vi "GetClassTemplateMethods.vi"(0 "MethodTemplatePath":path, 5 "error in":errorcluster) -> (6 "InterfaceMethodNames":string[](array[string]), 8 "InterfaceMethodPaths":path[](array[path]), 10 "NormalMethodNames":string[](array[string]), 11 "PropertyNodeMethodPaths":path[](array[path]), 12 "NormalMethodPaths":path[](array[path]), 13 "PropertyNodeMethodNames":string[](array[string]), 15 "OverrideMethodNames":string[](array[string]), 16 "OverrideMethodPaths":path[](array[path]), 17 "PropertyMethodNames":string[](array[string]), 18 "PropertyMethodPaths":path[](array[path]), 19 "error out":errorcluster)   [LabVIEW 2020, in "ClassWriterNative.lvclass"]
uses:
  <resource>/Framework/Providers/Open_GDS/ClassProviders/Provider_LvNativeClass/ClassWriterNative_class/ClassWriterNative.lvclass
  <vilib>/Utility/config.llb/Read Key (Path).vi
  <vilib>/Utility/config.llb/NI_LVConfig.lvlib
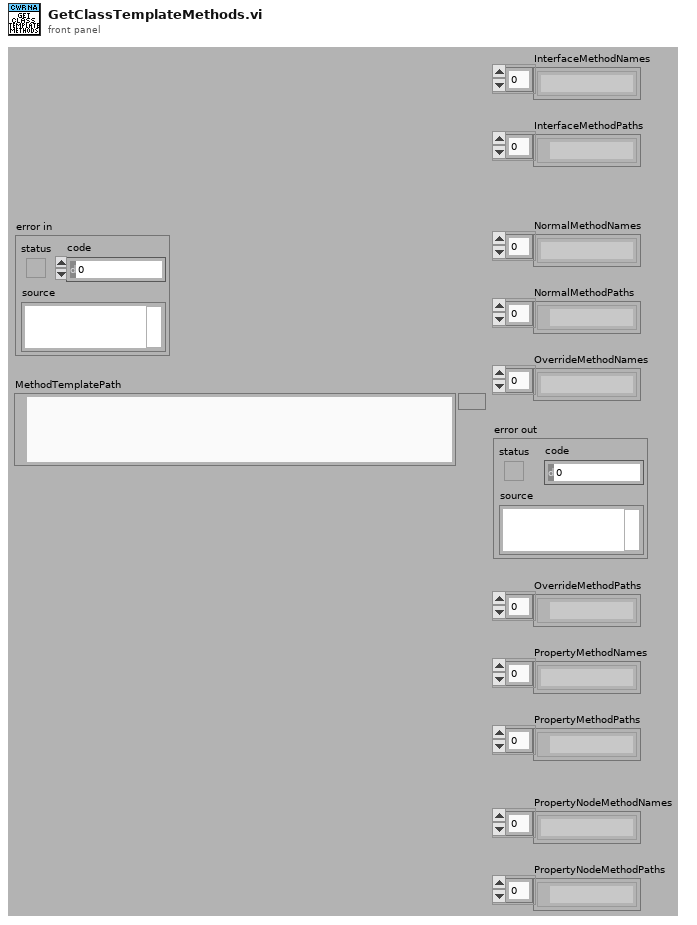
[diagram p1: front panel]
types:
  T1 = typedef "NI_LVConfig.lvlib/Config Data RefNum.ctl" = refnum<k1>
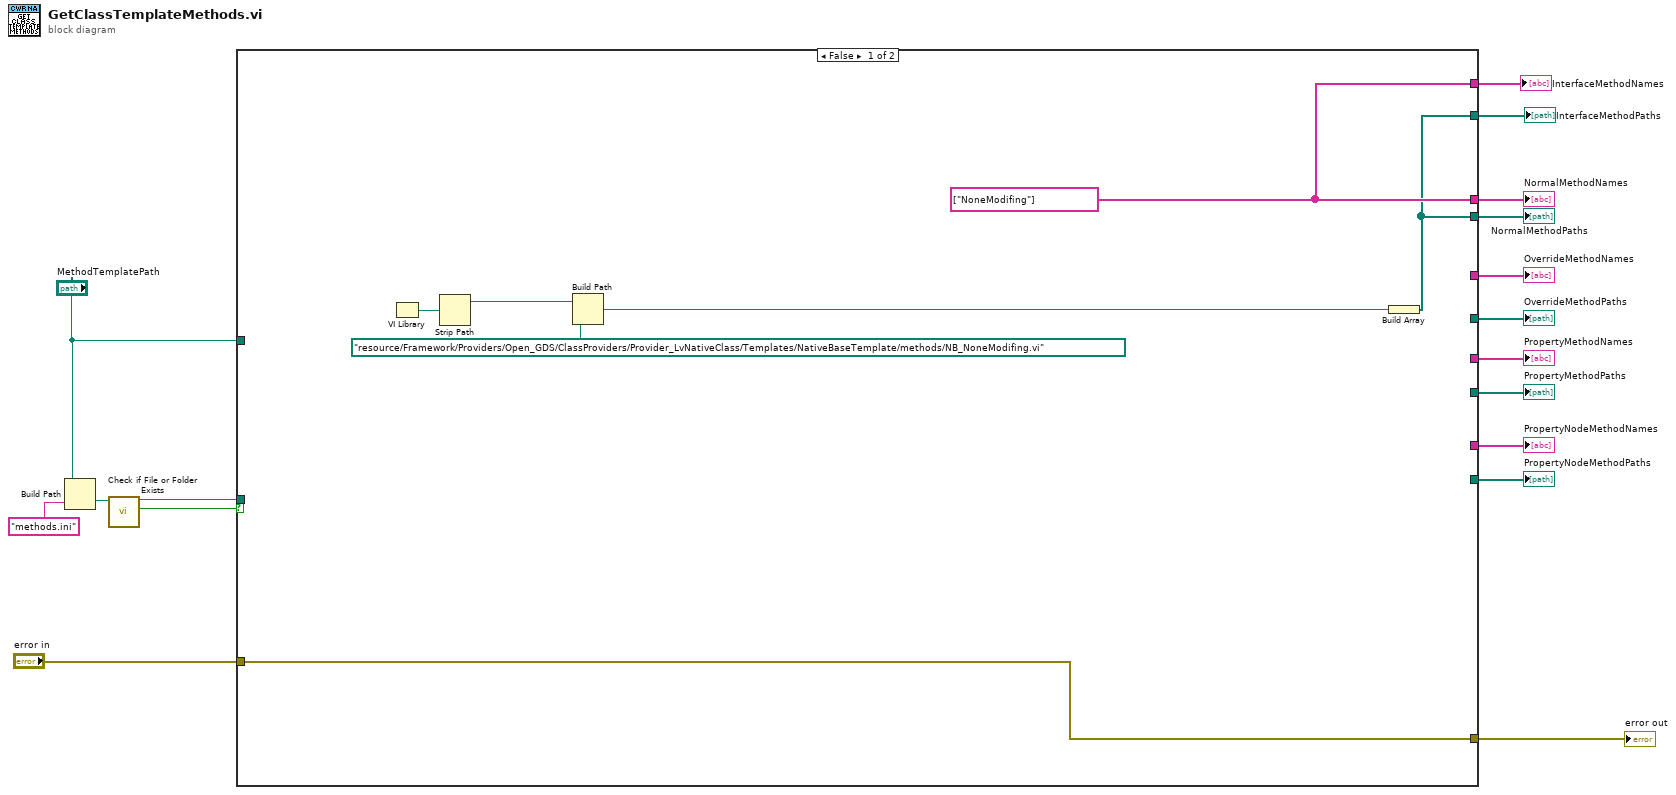
[diagram p0: block diagram]
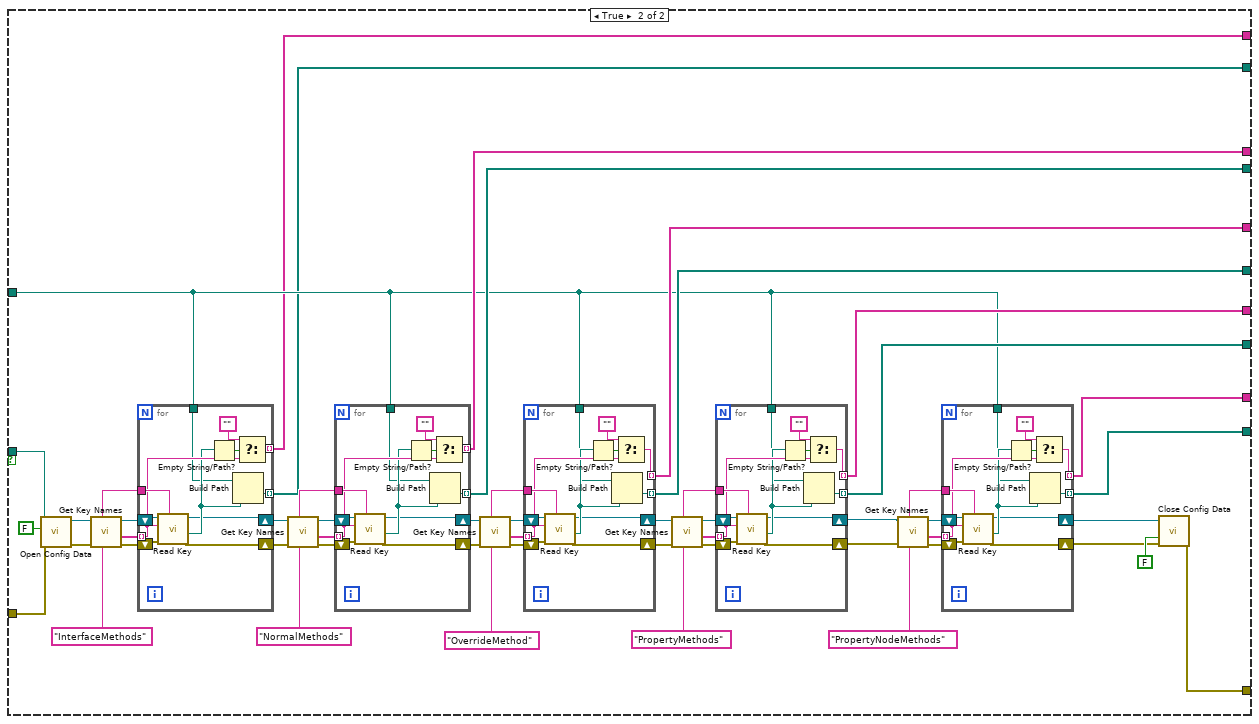
[diagram p2: hidden frame]
diagram:
  n1 = Build Path(base path="MethodTemplatePath", name or relative path="methods.ini") -> (appended path=w7:path)
  n2 = call <vilib>:"Check if File or Folder Exists.vi"("path"=w7) -> ("file or folder exists?"=w6:bool, "dup path"=w5:path)  [unwired: 8 in, 1 out]
  n3 = case shown="False" w6 {
    tunnel: "MethodTemplatePath" -> [_ w27]
    tunnel: [w18 w72] -> w16
    tunnel: "error in" -> [w24 w71]
    tunnel: [_ w68] -> w13
    tunnel: [_ w67] -> w12
    tunnel: [w19 w66] -> w11
    tunnel: [w24 w63] -> w10
    tunnel: [_ w62] -> w9
    tunnel: [_ w61] -> w8
    tunnel: w5 -> [_ w46]
    tunnel: [_ w36] -> w3
    tunnel: [_ w37] -> w4
    tunnel: [w19 w26] -> w2
    tunnel: [w18 w25] -> w1
    frame False {
      w19 = string[] ["NoneModifing"]
      n4 = VI Library() -> (path=w22:path)
      n5 = Strip Path(path=w22) -> (stripped path=w21:path)  [unwired: 1 out]
      n6 = Build Path(base path=w21, name or relative path=path "resource/Framework/Providers/Open_GDS/ClassProviders/Provider_LvNativeClass/Templates/NativeBaseTemplate/methods/NB_NoneModifing.vi" ("base path")) -> (appended path=w20:path)
      n7 = Build Array(w20) -> (w18:path[])
    }
    frame True {
      w33 = "InterfaceMethods" ("section")
      w38 = "PropertyNodeMethods" ("section")
      w70 = "OverrideMethod" ("section")
      w69 = "PropertyMethods" ("section")
      w49 = "NormalMethods" ("section")
      n8 = call <vilib>:"Open Config Data.vi"("error in (no error)"=w71, "create file if necessary (T)"=FALSE ("create file if necessary? (T)"), "configuration file path"=w46) -> ("error out"=w28:errorcluster, "refnum"=w29:T1)  [unwired: 6 in, 1 out]
      n9 = call <vilib>:"Get Key Names.vi"("section"=w33, "error in (no error)"=w28, "refnum"=w29) -> ("error out"=w35:errorcluster, "key names"=w32:string[], "refnum out"=w34:T1)  [unwired: 5 in, 1 out]
      n10 = for {
        shift-right: [w73] -> w31
        shift-left: w35 -> [w83]
        shift-right: [w74] -> w30
        shift-left: w34 -> [w84]
        tunnel: w33 -> [w82]
        tunnel: w32 -> [w80] mode=indexing
        tunnel: [w78] -> w26 mode=indexing
        tunnel: w27 -> [w76]
        tunnel: [w75] -> w25 mode=indexing
        n11 = call-poly <vilib>:"Read Key.vi"("section"=w82, "error in (no error)"=w83, "key"=w80, "refnum"=w84) -> ("error out"=w73:errorcluster, "value"=w77:path, "refnum out"=w74:T1)  [unwired: 4 in, 1 out]
        n12 = Empty String/Path?(string/path=w77) -> (empty?=w81:bool)
        n13 = Build Path(base path=w76, name or relative path=w77) -> (appended path=w75:path)
        n14 = Select(t="", s=w81, f=w80) -> (s? t:f=w78:string)
      }
      n15 = call <vilib>:"Get Key Names.vi"("section"=w49, "error in (no error)"=w31, "refnum"=w30) -> ("error out"=w47:errorcluster, "key names"=w50:string[], "refnum out"=w48:T1)  [unwired: 5 in, 1 out]
      n16 = for {
        shift-right: [w121] -> w52
        shift-left: w47 -> [w131]
        shift-right: [w122] -> w51
        shift-left: w48 -> [w132]
        tunnel: w49 -> [w130]
        tunnel: w50 -> [w128] mode=indexing
        tunnel: [w126] -> w66 mode=indexing
        tunnel: w27 -> [w124]
        tunnel: [w123] -> w72 mode=indexing
        n17 = call-poly <vilib>:"Read Key.vi"("section"=w130, "error in (no error)"=w131, "key"=w128, "refnum"=w132) -> ("error out"=w121:errorcluster, "value"=w125:path, "refnum out"=w122:T1)  [unwired: 4 in, 1 out]
        n18 = Empty String/Path?(string/path=w125) -> (empty?=w129:bool)
        n19 = Build Path(base path=w124, name or relative path=w125) -> (appended path=w123:path)
        n20 = Select(t="", s=w129, f=w128) -> (s? t:f=w126:string)
      }
      n21 = call <vilib>:"Get Key Names.vi"("section"=w70, "error in (no error)"=w52, "refnum"=w51) -> ("error out"=w53:errorcluster, "key names"=w55:string[], "refnum out"=w54:T1)  [unwired: 5 in, 1 out]
      n22 = for {
        shift-right: [w109] -> w59
        shift-left: w53 -> [w119]
        shift-right: [w110] -> w60
        shift-left: w54 -> [w120]
        tunnel: w70 -> [w118]
        tunnel: w55 -> [w116] mode=indexing
        tunnel: [w114] -> w67 mode=indexing
        tunnel: w27 -> [w112]
        tunnel: [w111] -> w68 mode=indexing
        n23 = call-poly <vilib>:"Read Key.vi"("section"=w118, "error in (no error)"=w119, "key"=w116, "refnum"=w120) -> ("error out"=w109:errorcluster, "value"=w113:path, "refnum out"=w110:T1)  [unwired: 4 in, 1 out]
        n24 = Empty String/Path?(string/path=w113) -> (empty?=w117:bool)
        n25 = Build Path(base path=w112, name or relative path=w113) -> (appended path=w111:path)
        n26 = Select(t="", s=w117, f=w116) -> (s? t:f=w114:string)
      }
      n27 = call <vilib>:"Get Key Names.vi"("section"=w69, "error in (no error)"=w59, "refnum"=w60) -> ("error out"=w58:errorcluster, "key names"=w56:string[], "refnum out"=w57:T1)  [unwired: 5 in, 1 out]
      n28 = for {
        shift-right: [w97] -> w41
        shift-left: w58 -> [w107]
        shift-right: [w98] -> w42
        shift-left: w57 -> [w108]
        tunnel: w69 -> [w106]
        tunnel: w56 -> [w104] mode=indexing
        tunnel: [w102] -> w61 mode=indexing
        tunnel: w27 -> [w100]
        tunnel: [w99] -> w62 mode=indexing
        n29 = call-poly <vilib>:"Read Key.vi"("section"=w106, "error in (no error)"=w107, "key"=w104, "refnum"=w108) -> ("error out"=w97:errorcluster, "value"=w101:path, "refnum out"=w98:T1)  [unwired: 4 in, 1 out]
        n30 = Empty String/Path?(string/path=w101) -> (empty?=w105:bool)
        n31 = Build Path(base path=w100, name or relative path=w101) -> (appended path=w99:path)
        n32 = Select(t="", s=w105, f=w104) -> (s? t:f=w102:string)
      }
      n33 = call <vilib>:"Get Key Names.vi"("section"=w38, "error in (no error)"=w41, "refnum"=w42) -> ("error out"=w43:errorcluster, "key names"=w45:string[], "refnum out"=w44:T1)  [unwired: 5 in, 1 out]
      n34 = for {
        shift-right: [w85] -> w39
        shift-left: w43 -> [w95]
        shift-right: [w86] -> w40
        shift-left: w44 -> [w96]
        tunnel: w38 -> [w94]
        tunnel: w45 -> [w92] mode=indexing
        tunnel: [w90] -> w37 mode=indexing
        tunnel: w27 -> [w88]
        tunnel: [w87] -> w36 mode=indexing
        n35 = call-poly <vilib>:"Read Key.vi"("section"=w94, "error in (no error)"=w95, "key"=w92, "refnum"=w96) -> ("error out"=w85:errorcluster, "value"=w89:path, "refnum out"=w86:T1)  [unwired: 4 in, 1 out]
        n36 = Empty String/Path?(string/path=w89) -> (empty?=w93:bool)
        n37 = Build Path(base path=w88, name or relative path=w89) -> (appended path=w87:path)
        n38 = Select(t="", s=w93, f=w92) -> (s? t:f=w90:string)
      }
      n39 = call <vilib>:"Close Config Data.vi"("error in (no error)"=w39, "write file if changed (T)"=FALSE ("create file if necessary? (T)"), "refnum"=w40) -> ("error out"=w63:errorcluster)  [unwired: 7 in, 1 out]
    }
  }
  "NormalMethodPaths" <- w16
  "OverrideMethodPaths" <- w13
  "OverrideMethodNames" <- w12
  "NormalMethodNames" <- w11
  "error out" <- w10
  "PropertyMethodPaths" <- w9
  "PropertyMethodNames" <- w8
  "PropertyNodeMethodPaths" <- w3
  "PropertyNodeMethodNames" <- w4
  "InterfaceMethodNames" <- w2
  "InterfaceMethodPaths" <- w1
